vi "FileCheck.vi"() -> (1 "파일수":u16, 2 "스톡스 파일 배열":string[](array[string]), 3 "안티스톡스 파일 배열":string[](array[string]), 5 "연결된 문자열":string)   [LabVIEW 2020]
panel:
  out "파일 이름":string[](array[string])
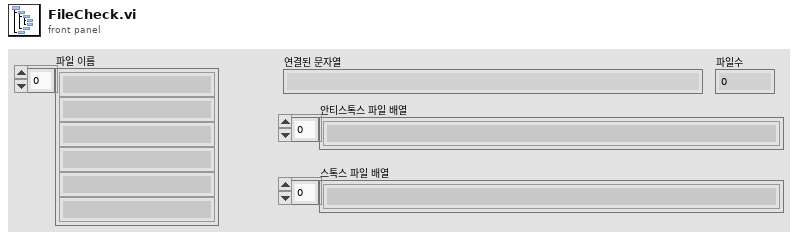
[diagram p1: front panel]
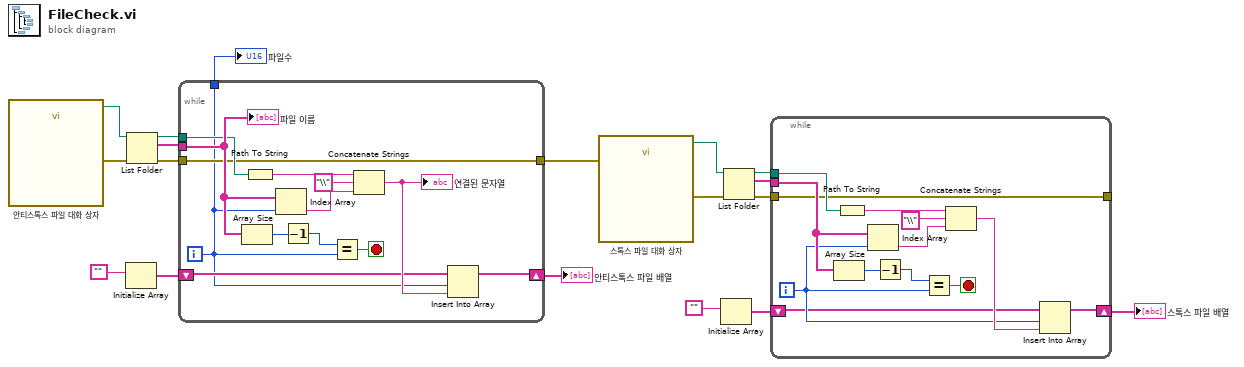
[diagram p0: block diagram]
diagram:
  n1 = call "안티스톡스 파일 대화 상자"() -> ("selected path"=w18:path, "error out"=w17:errorcluster)  [unwired: 12 in, 2 out]
  n2 = Initialize Array("") -> (w13:string[])  [unwired: 1 in]
  n3 = List Folder(path=w18, error in=w17) -> (path out=w16:path, filenames=w15:string[], error out=w11:errorcluster)  [unwired: 2 in, 1 out]
  n4 = while {
    tunnel: w16 -> [w23]
    tunnel: w15 -> [w27]
    shift-right: [w24] -> w12
    shift-left: w13 -> [w25]
    tunnel: [w22] -> w2
    tunnel: w11 -> [w22]
    tunnel: [w19] -> w1
    i -> [w19]
    stop <- w28 stop-if-true
    n5 = Array Size(array=w27) -> (size(s)=w31:i32)
    n6 = Path To String(path=w23) -> (string=w30:string)
    n7 = Index Array(array=w27, index=w19) -> (element=w21:string)
    n8 = Decrement(x=w31) -> (x-1=w29:i32)
    n9 = Equal?(x=w29, y=w19) -> (x = y?=w28:bool)
    n10 = Concatenate Strings(w30, "\\", w21) -> (w26:string)
    "연결된 문자열" <- w26
    n11 = Insert Into Array(array=w25, index=w19, new element=w26) -> (w24:string[])
    "파일 이름" <- w27
  }
  "안티스톡스 파일 배열" <- w12
  "파일수" <- w1
  n12 = call "스톡스 파일 대화 상자"("error in"=w2) -> ("selected path"=w10:path, "error out"=w9:errorcluster)  [unwired: 11 in, 2 out]
  n13 = Initialize Array("") -> (w5:string[])  [unwired: 1 in]
  n14 = List Folder(path=w10, error in=w9) -> (path out=w8:path, filenames=w7:string[], error out=w3:errorcluster)  [unwired: 2 in, 1 out]
  n15 = while {
    tunnel: w8 -> [w35]
    tunnel: w7 -> [w40]
    shift-right: [w36] -> w4
    shift-left: w5 -> [w37]
    tunnel: [w34] -> _
    tunnel: w3 -> [w34]
    i -> [w38]
    stop <- w41 stop-if-true
    n16 = Array Size(array=w40) -> (size(s)=w44:i32)
    n17 = Path To String(path=w35) -> (string=w43:string)
    n18 = Index Array(array=w40, index=w38) -> (element=w33:string)
    n19 = Decrement(x=w44) -> (x-1=w42:i32)
    n20 = Equal?(x=w42, y=w38) -> (x = y?=w41:bool)
    n21 = Concatenate Strings(w43, "\\", w33) -> (w39:string)
    n22 = Insert Into Array(array=w37, index=w38, new element=w39) -> (w36:string[])
  }
  "스톡스 파일 배열" <- w4
